vi "init runtime test.vi"() -> (0 "no error":errorcluster, 1 "tags found":bool, 2 "expected execution settings":bool)   [LabVIEW 2015, in "J1939 tests.lvlib"]
doc: "Tests the 'Initialize' VI of the module's runtime class."
uses:
  J1939 tests.lvlib
  module/execution/J1939 runtime.lvclass
  <vilib>/NI/Tag Bus/tag/tag descriptor.lvclass/tag descriptor.ctl
  <vilib>/NI/Tag Bus Module Framework/channel/TBM channel.lvclass/TBM channel.ctl
  <vilib>/NI/Tag Bus/tag/read tag name.vi
  <vilib>/NI/Tag Bus/tag/read data type.vi
  <vilib>/NI/Tag Bus Module Framework/channel/Read channel classification.vi
  module/configuration/J1939 configuration.lvclass
  <vilib>/NI/Tag Bus/dictionary/data dictionary.lvclass
  <vilib>/NI/Tag Bus Module Framework/channel/TBM channel.lvclass
panel:
  out "Array":errorcluster[](array[cluster])
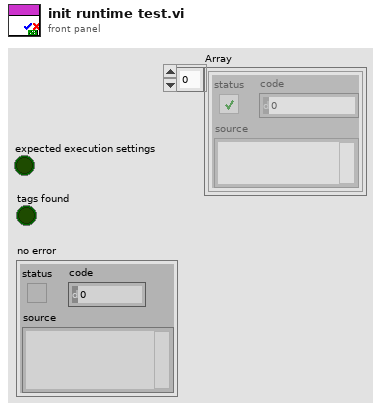
[diagram p1: front panel]
types:
  T1 = typedef "TBM channel.lvclass/data tables.ctl" = cluster{"input data":T2, "processing parameter":T2, "processing result":T2, "output data":T2}
  T2 = typedef "tag bus.lvlib/dictionary table pair.ctl" = cluster{"data dictionary":refnum<class "data dictionary.lvclass">, "data table":T3}
  T3 = typedef "tag bus.lvlib/data table.lvlib/data table.ctl" = cluster{"Double":dbl[], "Single":sgl[], "I64":i64[], "I32":i32[], "I16":i16[], "I8":i8[], "U64":u64[], "U32":u32[], "U16":u16[], "U8":u8[], "Boolean":bool[], "String":string[], "Array of Double":cluster{"DBL Array":dbl[]}[], "Array of Single":cluster{"SGL Array":sgl[]}[], "Array of I64":cluster{"I64 Array":i64[]}[], "Array of I32":cluster{"I32 Array":i32[]}[], "Array of I16":cluster{"I16 Array":i16[]}[], "Array of I8":cluster{"I8 Array":i8[]}[], "Array of U64":cluster{"U64 Array":u64[]}[], "Array of U32":cluster{"U32 Array":u32[]}[], "Array of U16":cluster{"U16 Array":u16[]}[], "Array of U8":cluster{"U8 Array":u8[]}[], "Array of Boolean":cluster{"Boolean Array":bool[]}[], "Array of String":cluster{"String Array":string[]}[]}
  T4 = typedef "TBM module execution interface.lvclass/execution settings.ctl" = cluster{"reads inputs":bool, "processes data":bool, "writes outputs":bool}
  T5 = typedef "tag bus.lvlib/tag descriptor.lvclass/Data Type.ctl" = enum16{"Double", "Single", "I64", "I32", "I16", "I8", "U64", "U32", "U16", "U8", "Boolean", "String", "Array of Double", "Array of Single", "Array of I64", "Array of I32", "Array of I16", "Array of I8", "Array of U64", "Array of U32", "Array of U16", "Array of U8", "Array of Boolean", "Array of String"}
  T6 = typedef "TBM channel.lvclass/channel classification.ctl" = enum16{"input data", "output data", "processing parameter", "processing result"}
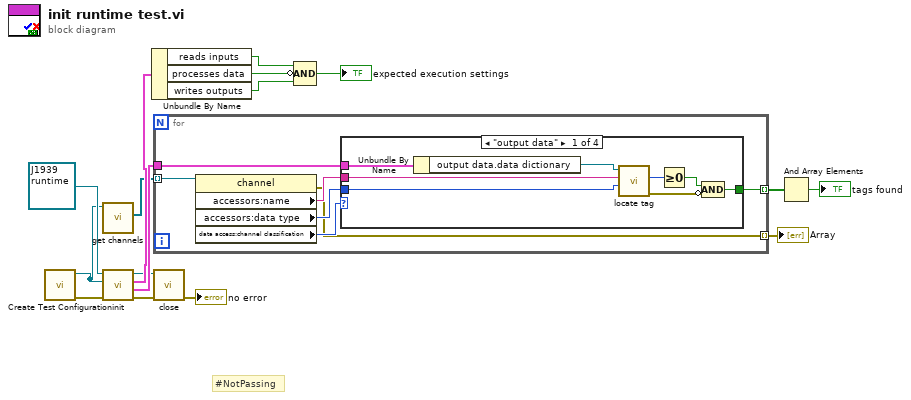
[diagram p0: block diagram]
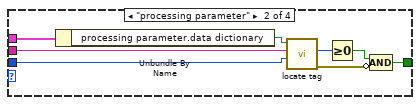
[diagram p2: hidden frame]
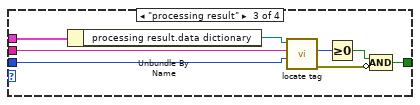
[diagram p3: hidden frame]
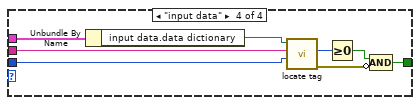
[diagram p4: hidden frame]
diagram:
  # "#NotPassing"
  n1 = call "Create Test Configuration.vi"() -> ("error out"=w4:errorcluster, "Module Configuration"=w3:refnum<class "J1939 configuration.lvclass">)  [unwired: 5 in, 5 out]
  n2 = call-dynamic "get channels.vi"("J1939 configuration in"=w3) -> ("channels"=w2:refnum<class "TBM channel.lvclass">[])  [unwired: 9 in, 1 out]
  n3 = call-dynamic "init.vi"("error in"=w4, "TBM module configuration in"=w3, "J1939 runtime in"=refnum<class "J1939 runtime.lvclass"> refnum ("tag bus configurable plugin module")) -> ("error out"=w8:errorcluster, "data allocations"=w16:T1, "execution settings"=w15:T4, "J1939 runtime out"=w7:refnum<class "J1939 runtime.lvclass">)  [unwired: 5 in]
  n4 = Unbundle By Name(w15) -> ("reads inputs"=w14:bool, "processes data"=w12:bool, "writes outputs"=w13:bool)
  n5 = for {
    tunnel: w16 -> [w23]
    tunnel: w2 -> [w22] mode=indexing
    tunnel: [w21] -> w10 mode=indexing
    tunnel: [w17] -> w1 mode=indexing
    n6 = property class="channel"(reference=w22) -> (error out=w17:errorcluster, "accessors:name"=w18:string, "accessors:data type"=w19:T5, "data access:channel classification"=w20:T6)  [unwired: 1 in, 1 out]
    n7 = case shown="\"output data\"" w20 {
      tunnel: w23 -> [w31 w39 w47 w55]
      tunnel: w19 -> [w29 w37 w45 w53]
      tunnel: w18 -> [w28 w36 w44 w52]
      tunnel: [w24 w32 w40 w48] -> w21
      frame "output data" {
        n8 = Unbundle By Name(w31) -> ("output data.data dictionary"=w30:refnum<class "data dictionary.lvclass">)
        n9 = call <vilib>:"locate tag.vi"("data type"=w29, "name"=w28, "data dictionary in"=w30) -> ("error out"=w25:errorcluster, "index"=w27:i32)  [unwired: 6 in, 1 out]
        n10 = Greater Or Equal To 0?(x=w27) -> (x >= 0?=w26:bool)
        n11 = Compound Arithmetic op=AND(w26, invert w25) -> (w24:bool)
      }
      frame "processing parameter" {
        n12 = Unbundle By Name(w39) -> ("processing parameter.data dictionary"=w38:refnum<class "data dictionary.lvclass">)
        n13 = call <vilib>:"locate tag.vi"("data type"=w37, "name"=w36, "data dictionary in"=w38) -> ("error out"=w33:errorcluster, "index"=w35:i32)  [unwired: 6 in, 1 out]
        n14 = Greater Or Equal To 0?(x=w35) -> (x >= 0?=w34:bool)
        n15 = Compound Arithmetic op=AND(w34, invert w33) -> (w32:bool)
      }
      frame "processing result" {
        n16 = Unbundle By Name(w47) -> ("processing result.data dictionary"=w46:refnum<class "data dictionary.lvclass">)
        n17 = call <vilib>:"locate tag.vi"("data type"=w45, "name"=w44, "data dictionary in"=w46) -> ("error out"=w41:errorcluster, "index"=w43:i32)  [unwired: 6 in, 1 out]
        n18 = Greater Or Equal To 0?(x=w43) -> (x >= 0?=w42:bool)
        n19 = Compound Arithmetic op=AND(w42, invert w41) -> (w40:bool)
      }
      frame "input data" {
        n20 = Unbundle By Name(w55) -> ("input data.data dictionary"=w54:refnum<class "data dictionary.lvclass">)
        n21 = call <vilib>:"locate tag.vi"("data type"=w53, "name"=w52, "data dictionary in"=w54) -> ("error out"=w49:errorcluster, "index"=w51:i32)  [unwired: 6 in, 1 out]
        n22 = Greater Or Equal To 0?(x=w51) -> (x >= 0?=w50:bool)
        n23 = Compound Arithmetic op=AND(w50, invert w49) -> (w48:bool)
      }
    }
  }
  "Array" <- w1
  n24 = call-dynamic "close.vi"("error in"=w8, "J1939 runtime in"=w7) -> ("error out"=→"no error":errorcluster)  [unwired: 9 in]
  n25 = Compound Arithmetic op=AND(w14, invert w12, w13) -> (→"expected execution settings":bool)
  n26 = And Array Elements(Boolean array=w10) -> (logical AND=→"tags found":bool)
